vi "Sync_triggers.vi"(0 "PRP":u32, 2 "Pulse width":u16, 3 "Guard width":u16) -> (1 "no_guard":bool, 4 "end_Rx":bool, 6 "start_Tx":bool, 7 "end_Tx":bool, 8 "start_Rx":bool)   [LabVIEW 2017]
uses:
  <vilib>/rvi/FXPMathLib/basic elements/FxpDiscreteDelay/XNode/nifxpmath_DiscreteDelay.xnode
panel:
  out "count_prp":u32
  out "count_pulse":u16
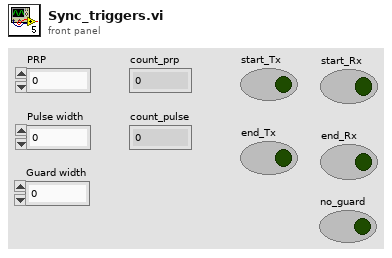
[diagram p1: front panel]
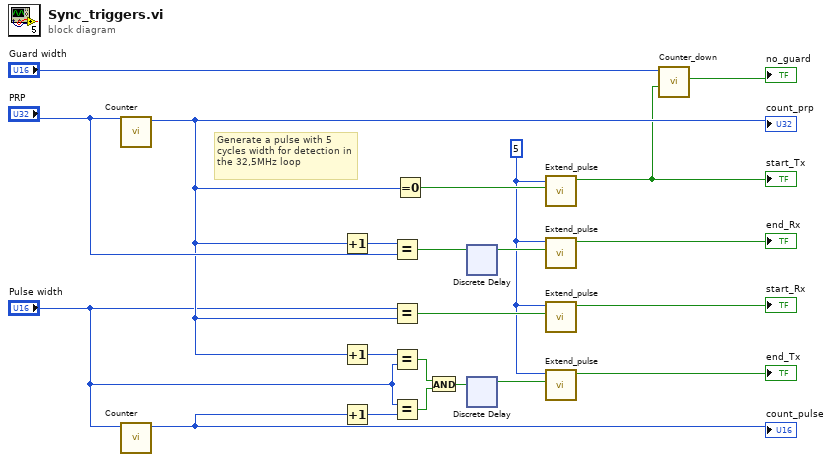
[diagram p0: block diagram]
diagram:
  w3 = u16 5 ("limit")
  # "Generate a pulse with 5 cycles width for detection in the 32,5MHz loop"
  n1 = call "Counter.vi"("limit"="PRP") -> ("count"=w18:u32)  [unwired: 9 in, 1 out]
  "count_prp" <- w18
  n2 = call "Counter.vi"("limit"="Pulse width") -> ("count"=w21:u32)  [unwired: 9 in, 1 out]
  "count_pulse" <- w21
  n3 = Increment(x=w18) -> (x+1=w11:u32)
  n4 = Increment(x=w18) -> (x+1=w6:u32)
  n5 = Increment(x=w21) -> (x+1=w4:u32)
  n6 = Equal?(x=w11, y="PRP") -> (x = y?=w19:bool)
  n7 = Equal?(x="Pulse width", y=w18) -> (x = y?=w12:bool)
  n8 = Equal?(x=w6, y="Pulse width") -> (x = y?=w8:bool)
  n9 = Equal?(x="Pulse width", y=w4) -> (x = y?=w7:bool)
  n10 = Equal To 0?(x=w18) -> (x = 0?=w13:bool)
  n11 = And(x=w8, y=w7) -> (x .and. y?=w20:bool)
  n12 = xnode ("Discrete Delay")("D"=w19) -> ("Q"=w15:bool)
  n13 = xnode ("Discrete Delay")("D"=w20) -> ("Q"=w17:bool)
  n14 = call "Extend_pulse.vi"("reset"=w13, "limit"=w3) -> ("pulse"=w1:bool)  [unwired: 9 in]
  "start_Tx" <- w1
  n15 = call "Extend_pulse.vi"("reset"=w15, "limit"=w3) -> ("pulse"=→"end_Rx":bool)  [unwired: 9 in]
  n16 = call "Extend_pulse.vi"("reset"=w12, "limit"=w3) -> ("pulse"=→"start_Rx":bool)  [unwired: 9 in]
  n17 = call "Extend_pulse.vi"("reset"=w17, "limit"=w3) -> ("pulse"=→"end_Tx":bool)  [unwired: 9 in]
  n18 = call "Counter_down.vi"("load"=w1, "limit"="Guard width") -> ("count = 0?"=→"no_guard":bool)  [unwired: 8 in, 1 out]
